vi "Measure_Synthetic_Jet.vi"(3 "Mode":T1=enum."Run VI", 5 "Traverse line In":T3={"Start X"=0.0, "Start Y"=0.0, "Start Z"=0.0, "End X"=nan, "End Y"=nan, "End Z"=nan, "No. of pts."=5, "Spacing"=enum."Linear", "Filename"=path "C:/EnFlo_Data_Local/2013/Aero_Tunnel/Nick_Martin/Results/01-2013/QA_test_I.xls", "Tunnel Speed"=nan, "Averaging time (min)"=0.08, "Extra Commands"="", "Specific Arguments"="Measure_Synthetic_Jet.vi; 200; 1000; 100", "Emission Rate (l/min)"=nan, "Trace Gas Concentration (%)"=nan, "Density Ratio"="  ---------", "Comments"="", "Row No"=0, "Row Type Selector"=enum."Run VI Named:", "Completion time"="17:12  07-01-2013", "Row Duration (mins)"=4.483248000000001, "No. of Valid pts."=5, "Meas Setup File"="LDA_SJ_A.xls"} {"Row Duration (mins)" format="%#.1f"; "Row No" min=0; "Trace Gas Concentration (%)" min=0.0 format="%#.2f"; "Emission Rate (l/min)" format="%#.2f"; "Tunnel Speed" format="%#.2f"; "Start X" format="%#.2f"; "Start Y" format="%#.2f"; "Start Z" format="%#.2f"; "End X" format="%#.2f"; "End Y" format="%#.2f"; "End Z" format="%#.2f"; "Averaging time (min)" min=0.0 format="%#.2f"}) -> (0 "Error Message":string, 1 "Status":T2, 2 "Traverse line Out":T3={"Start X"=0.0, "Start Y"=0.0, "Start Z"=0.0, "End X"=nan, "End Y"=nan, "End Z"=nan, "No. of pts."=5, "Spacing"=enum."Linear", "Filename"=path "C:/EnFlo_Data_Local/2013/Aero_Tunnel/Nick_Martin/Results/01-2013/QA_test_I.xls", "Tunnel Speed"=nan, "Averaging time (min)"=0.08, "Extra Commands"="", "Specific Arguments"="Measure_Synthetic_Jet.vi; 200; 1000; 100", "Emission Rate (l/min)"=nan, "Trace Gas Concentration (%)"=nan, "Density Ratio"="  ---------", "Comments"="", "Row No"=0, "Row Type Selector"=enum."Run VI Named:", "Completion time"="17:12  07-01-2013", "Row Duration (mins)"=4.483248000000001, "No. of Valid pts."=5, "Meas Setup File"="LDA_SJ_A.xls"} {"Row Duration (mins)" format="%#.1f"; "Row No" min=0; "Trace Gas Concentration (%)" min=0.0 format="%#.2f"; "Emission Rate (l/min)" format="%#.2f"; "Tunnel Speed" format="%#.2f"; "Start X" format="%#.2f"; "Start Y" format="%#.2f"; "Start Z" format="%#.2f"; "End X" format="%#.2f"; "End Y" format="%#.2f"; "End Z" format="%#.2f"; "Averaging time (min)" min=0.0 format="%#.2f"})   [LabVIEW 2012]
uses:
  Gen Trav/Traverse_cluster.ctl
  Gen Trav/Spacing.ctl
  Controls/Multi_run_mode.ctl
  Gen Trav/Multi_Run_Status.ctl
  Controls/User_Specific_mode.ctl
  Controls/Setup.ctl
  Controls/Save_Data.ctl
  ADAM Client/Sub VIs/ADAM Controls/Update_scan_value.ctl
  Globals/Meas_global.vi
  Globals/Synthetic_jet_global.vi
  <vilib>/Analysis/1siggen.llb/Ramp Pattern by Samples.vi
  Globals/Extra_Commands_Global.vi
  <vilib>/Analysis/NI_AALBase.lvlib
panel:
  in  "Enter SJ Data?":bool=TRUE
  in  "Stop Button":bool
  out "Last Meas Point":bool=TRUE
  out "Data":cluster{"Ramp Pattern":dbl[], dbl[]}[](graph)
  in  "Channels to Analyse":i32[](listbox)=[0]
  in  "VISA resource name":refnum<visa-resource-name>="USB0::0x0699::0x0347::C036837::INSTR"
  out "First Meas Point":bool=TRUE
  # "Check the Multirun in order to populate these Channels!"
  # "X           Y            Z"
  # "Start"
  # "End"
  # "X           Y            Z"
  # "Start"
  # "End"
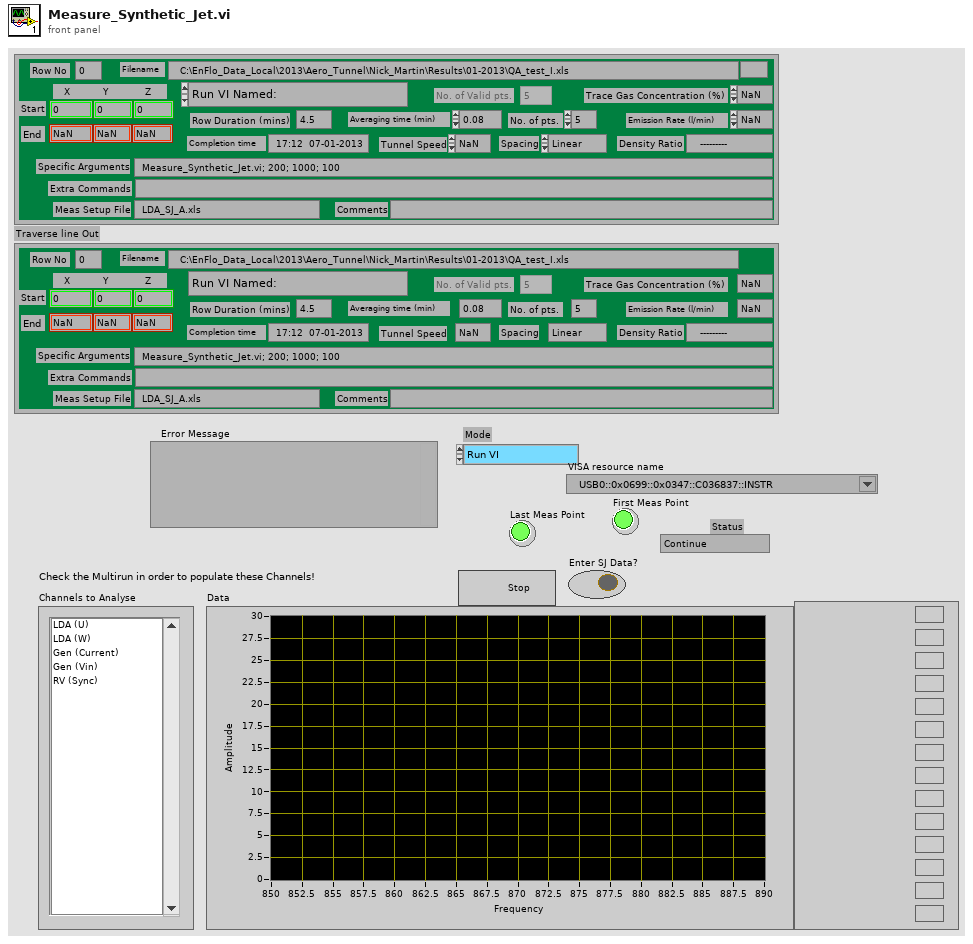
[diagram p1: front panel]
types:
  T1 = typedef "User_Specific_mode.ctl" = enum16{"Check VI only", "Run VI"}
  T2 = typedef "Multi_Run_Status.ctl" = enum16{"Continue", "Jump to Next Point", "Jump to Next Row", "Jump To Fall Back", "Terminate Run"}
  T3 = typedef "Traverse_cluster.ctl" = cluster{"Start X":dbl, "Start Y":dbl, "Start Z":dbl, "End X":dbl, "End Y":dbl, "End Z":dbl, "No. of pts.":i32, "Spacing":T4, "Filename":path, "Tunnel Speed":dbl, "Averaging time (min)":dbl, "Extra Commands":string, "Specific Arguments":string, "Emission Rate (l/min)":dbl, "Trace Gas Concentration (%)":dbl, "Density Ratio":string, "Comments":string, "Row No":i32, "Row Type Selector":T5, "Completion time":string, "Row Duration (mins)":dbl, "No. of Valid pts.":i32, "Meas Setup File":string}
  T4 = typedef "Spacing.ctl" = enum16{"Linear", "Log", "Gauss", "Specified", "N/A"}
  T5 = typedef "Multi_run_mode.ctl" = enum16{"Move Traverse Only", "Set Tunnel Speed Only", "Set Source Only", "Set Measurement Conditions", "Single Measurement", "Vertical Profile", "Lateral Profile", "Longitudinal Profile", "Explore Volume", "Multi-Axis Profile", "Auto Calibrate", "Meas Fast FID Bkgnd", "Check Beam Power", "Scanning Valve Measurement", "Run VI Named:", "Set ADAM Ch", "Wait (minutes)", "Send Message", "Synchronize With:", "Fall Back to this Row", "Turn Off Row Repeating", "Blank Row", "Traverse 3D Volume"}
  T6 = typedef "Analysis_info_cluster.ctl" = cluster{"Colour":u32, "Inst type":T7, "Inst name":string, "Symbol":string, "Code name":string, "Extra Info":string, "Inst Array":T8, "Extra Titles":string[], "Extra Values":string[], "U":dbl, "u^2":dbl, "u^3":dbl, "u^4":dbl, "Skew_u":dbl, "Kurt_u":dbl, "Sd Error in Mean":dbl, "% u'/U":dbl, "X":dbl, "Y":dbl, "Z":dbl, "Timescale integral to 25%":dbl, "Sd Error in Variance":dbl, "Calib File":path, "Calib Constants":dbl[], "Output Position":bool, "Full Stats":bool, "Av Sampling Rate":dbl, "Av No of Samples":dbl, "Total Meas Time (s)":dbl, "ADAM Ch Name":string}
  T7 = typedef "Inst_type.ctl" = enum16{"Propeller anemometer", "Raw voltage", "Pressure Transducer", "Pitot-static tube", "Preston tube", "Hot wire", "Cross wire 1", "Cross wire 2", "Generic Linear", "Generic Polynomial", "Generic BackPoly", "Fast FID", "Thermocouple", "Cold wire", "Pulsed Wire", "LDA Vel", "LDA Tran time", "LDA Arr time"}
  T8 = typedef "Instrument_Array.ctl" = enum16{"PWA", "LDA", "Analogue"}
  T9 = typedef "Save_Data.ctl" = enum16{"Save No Data", "Save Data"}
  T10 = typedef "Setup.ctl" = enum16{"Run Program", "Show Setup", "Save Current Setup", "Setup Front Panel"}
  T11 = typedef "SJ_Data_Cluster.ctl" = cluster{"Do (mm)":dbl, "Dc (mm)":dbl, "Ho (mm)":dbl, "Hc (mm)":dbl, "K":dbl, "beta":dbl, "Vc (m^3)":dbl, "Vo (m^3)":dbl}
  T12 = typedef "Update_scan_value.ctl" = cluster{"Channel Name":string, "New Value":dbl}
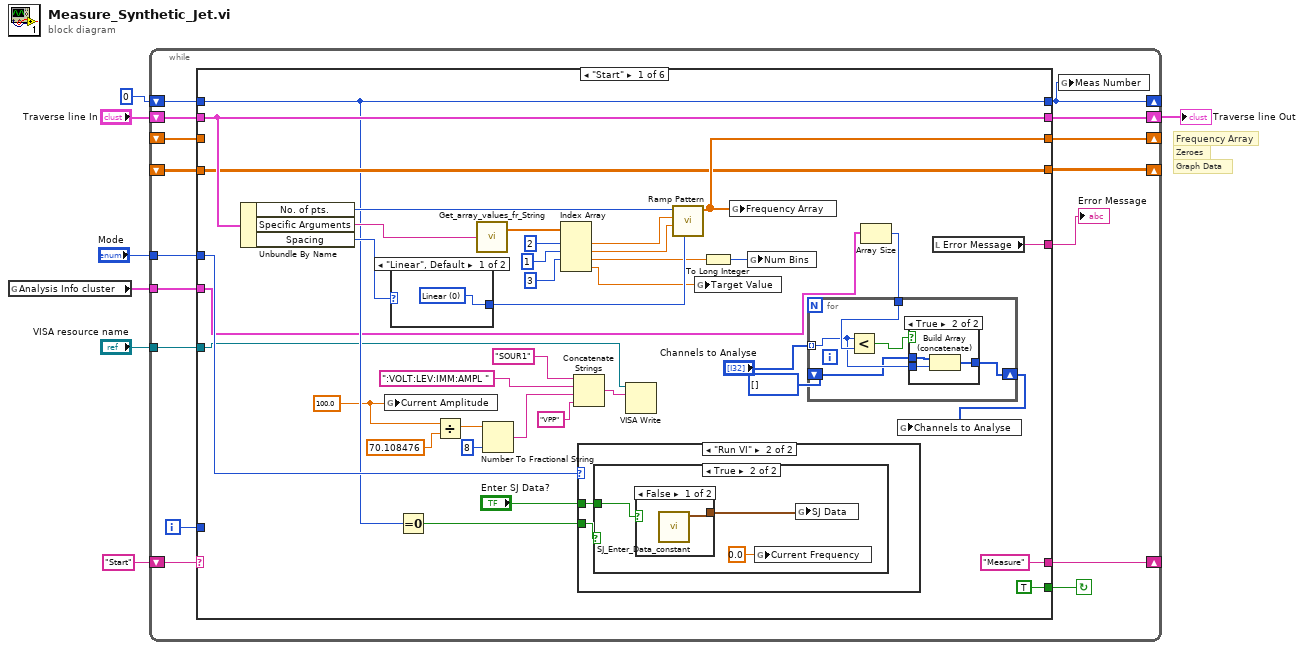
[diagram p0: block diagram]
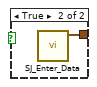
[diagram p5: hidden frame]
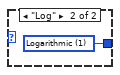
[diagram p6: hidden frame]
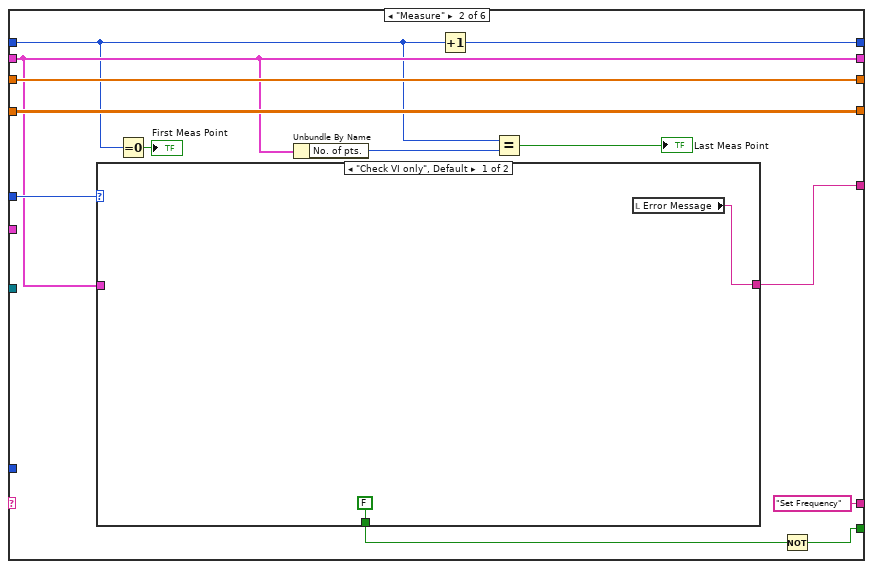
[diagram p7: hidden frame]
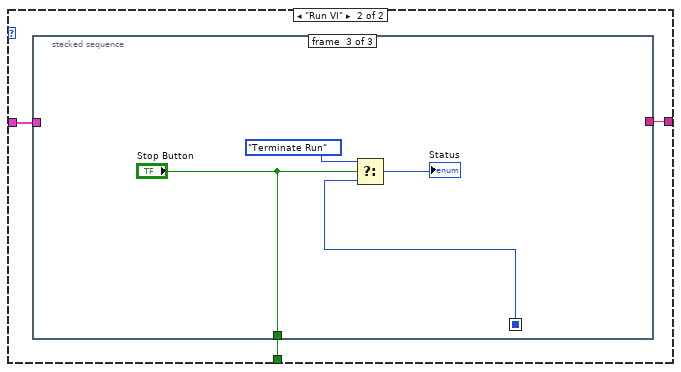
[diagram p8: hidden frame]
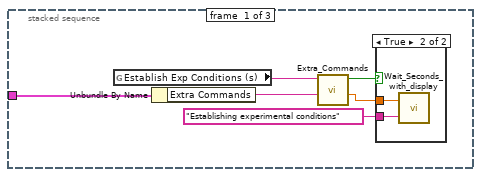
[diagram p9: hidden frame]
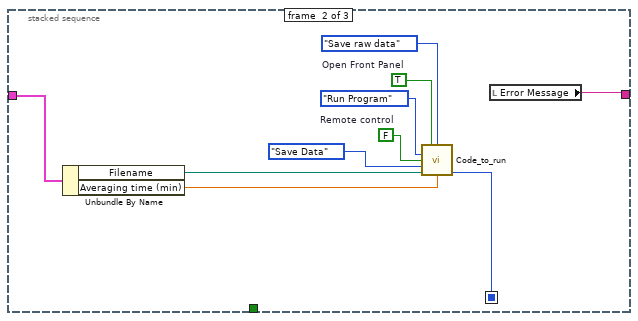
[diagram p11: hidden frame]
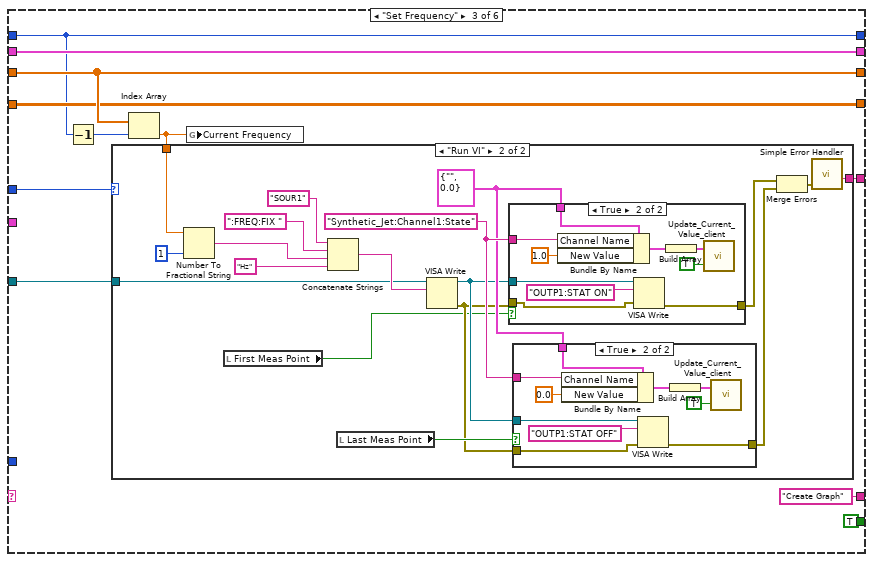
[diagram p12: hidden frame]
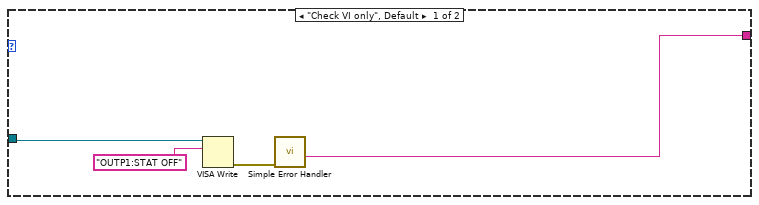
[diagram p13: hidden frame]
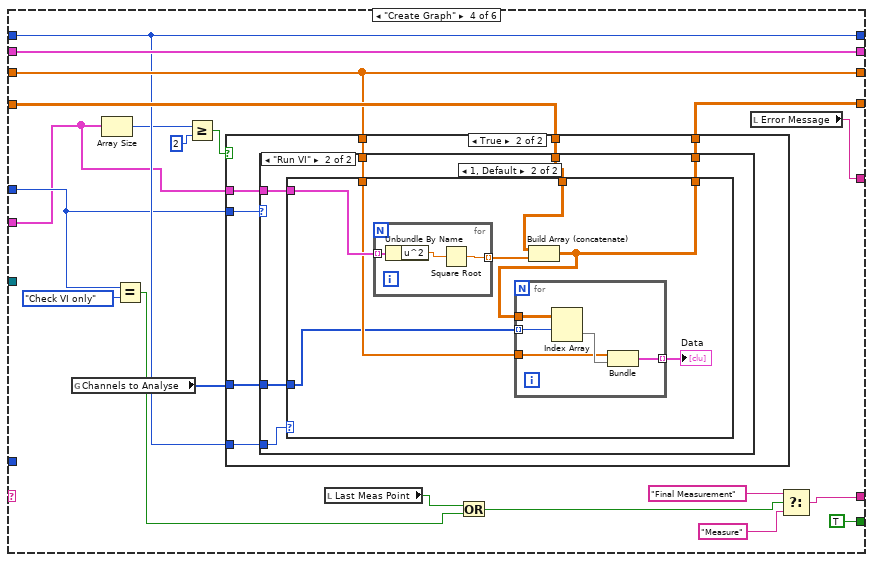
[diagram p16: hidden frame]
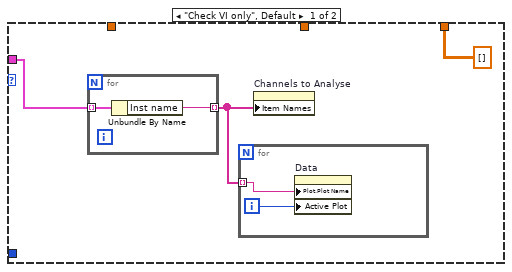
[diagram p18: hidden frame]
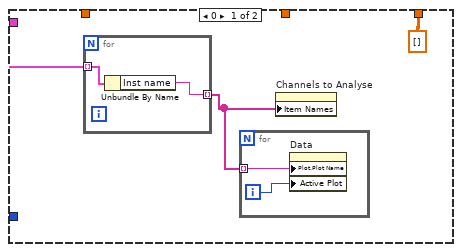
[diagram p19: hidden frame]
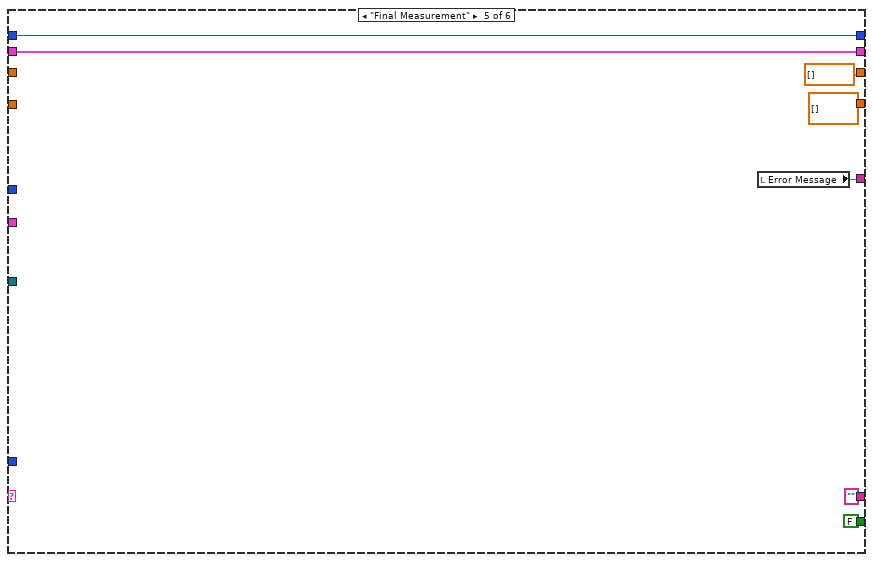
[diagram p20: hidden frame]
diagram:
  # "Graph Data"
  # "Zeroes"
  # "Frequency Array"
  n1 = global read "Meas_global.vi" "Analysis Info cluster"() -> (w1:T6[])
  n2 = while {
    shift-right: [w21] -> _
    shift-left: "Start" -> [w20]
    shift-right: [w19] -> w5
    shift-left: "Traverse line In" -> [w23]
    shift-right: [w18] -> _
    shift-left: _ -> [w17]
    tunnel: "Mode" -> [w16]
    tunnel: "VISA resource name" -> [w14]
    shift-right: [w13] -> _
    shift-left: _ -> [w12]
    shift-right: [w9] -> _
    shift-left: 0 -> [w10]
    tunnel: w1 -> [w8]
    i -> [w15]
    stop <- w22 continue-if-true
    n3 = case shown="\"Start\"" w20 {
      selector: w20 -> [_ _ _ _ _ w249]
      tunnel: w23 -> [w59 w86 w128 w194 w242 w257]
      tunnel: [TRUE w80 TRUE TRUE ("Last Meas Point") FALSE ("Last Meas Point") FALSE] -> w22
      tunnel: ["Measure" "Set Frequency" "Create Graph" w188 "" ""] -> w21
      tunnel: [w59 w86 w128 w194 w242 w257] -> w19
      tunnel: [w47 w91 w127 w191 dbl[] [] ("Ramp Pattern") w248] -> w18
      tunnel: w17 -> [_ w91 w127 w191 _ w248]
      tunnel: w16 -> [w48 w90 w123 w184 _ _]
      tunnel: w15 -> [_ _ _ _ _ _]
      tunnel: w14 -> [w33 _ w124 _ _ _]
      tunnel: [w46 w89 w122 w193 dbl[][] [] w247] -> w13
      tunnel: w12 -> [w46 w89 w122 w192 _ w247]
      tunnel: [w45 w88 w121 w190 w241 w246] -> w11
      tunnel: [w41 w84 w120 w185 w238 w245] -> w9
      tunnel: w10 -> [w41 w82 w120 w185 w238 w245]
      tunnel: w8 -> [w28 _ _ w175 _ _]
      frame "Start" {
        w30 = 100.0 ("number")
        n4 = Unbundle By Name(w59) -> ("No. of pts."=w58:i32, "Specific Arguments"=w55:string, "Spacing"=w57:T4)
        n5 = global write "Synthetic_jet_global.vi" "Current Amplitude"(w30) -> ()
        n6 = case shown="\"Linear\", Default" w57 {
          tunnel: [w78 w79] -> w56
          frame "Linear", Default {
            w78 = u16 0 items=["Linear", "Logarithmic"] ("type")
          }
          frame "Log" {
            w79 = u16 1 items=["Linear", "Logarithmic"] ("type")
          }
        }
        n7 = Equal To 0?(x=w41) -> (x = 0?=w49:bool)
        n8 = Divide(x=w30, y=70.108476) -> (x/y=w32:dbl)
        n9 = call "Get_array_values_fr_String.vi"("String Value"=w55) -> ("Numeric Array"=w54:dbl[])  [unwired: 1 out]
        n10 = Number To Fractional String(number=w32, precision (6)=i16 8) -> (F-format string=w35:string)  [unwired: 2 in]
        n11 = Index Array(array=w54, index #1=2 ("index"), index #2=1 ("index"), index #3=3 ("index")) -> (element #1=w51:dbl, element #2=w50:dbl, element #3=w43:dbl, element #4=w40:dbl)  [unwired: 1 in]
        n12 = Concatenate Strings("SOUR1" ("string"), ":VOLT:LEV:IMM:AMPL " ("string"), w35, "VPP" ("string")) -> (w36:string)
        n13 = case shown="\"Run VI\"" w48 {
          tunnel: w49 -> [_ w72]
          tunnel: "Enter SJ Data?" -> [_ w71]
          frame "Check VI only", Default {
          }
          frame "Run VI" {
            n14 = case shown="True" w72 {
              tunnel: w71 -> [_ w74]
              frame False {
              }
              frame True {
                n15 = case shown="False" w74 {
                  tunnel: [w76 w77] -> w73
                  frame False {
                    n16 = call "SJ_Enter_Data_constant.vi"() -> ("SJ Data"=w76:T11)  [unwired: 11 in]
                  }
                  frame True {
                    n17 = call "SJ_Enter_Data.vi"() -> ("SJ Data"=w77:T11)  [unwired: 11 in]
                  }
                }
                n18 = global write "Synthetic_jet_global.vi" "Current Frequency"(0.0 ("Current Frequency")) -> ()
                n19 = global write "Synthetic_jet_global.vi" "SJ Data"(w73) -> ()
              }
            }
          }
        }
        n20 = VISA Write(VISA resource name=w33, write buffer=w36) -> ()  [unwired: 1 in, 3 out]
        n21 = call-poly <vilib>:"Ramp Pattern.vi"("type"=w56, "start"=w50, "end"=w51, "samples"=w58) -> ("Ramp Pattern"=w47:dbl[])  [unwired: 6 in, 1 out]
        n22 = global write "Synthetic_jet_global.vi" "Target Value"(w40) -> ()
        n23 = To Long Integer(number=w43) -> (32bit integer=w42:i32)
        n24 = global write "Synthetic_jet_global.vi" "Frequency Array"(w47) -> ()
        n25 = global write "Synthetic_jet_global.vi" "Num Bins"(w42) -> ()
        n26 = Array Size(array=w28) -> (size(s)=w29:i32)
        n27 = for {
          tunnel: w29 -> [w66]
          tunnel: "Channels to Analyse" -> [w64] mode=indexing
          shift-right: [w63] -> w26
          shift-left: i32[] [] -> [w62]
          n28 = Less?(x=w64, y=w66) -> (x < y?=w65:bool)
          n29 = case shown="True" w65 {
            tunnel: w64 -> [_ w70]
            tunnel: [w67 w69] -> w63
            tunnel: w62 -> [w67 w68]
            frame False {
            }
            frame True {
              n30 = Build Array (concatenate)(w68, w70) -> (w69:i32[])
            }
          }
        }
        n31 = global write "Synthetic_jet_global.vi" "Channels to Analyse"(w26) -> ()
        n32 = local read "Error Message"() -> (w45:string)
      }
      frame "Measure" {
        n33 = case shown="\"Check VI only\", Default" w90 {
          tunnel: w86 -> [_ w97]
          tunnel: [w94 w96] -> w88
          tunnel: [FALSE ("Stop Button") w95] -> w81
          frame "Check VI only", Default {
            n34 = local read "Error Message"() -> (w94:string)
          }
          frame "Run VI" {
            n35 = stacked-sequence {
              seq-local: [_ w106 _] -> [_ _ w117]
              tunnel: w97 -> [w98 w111 _]
              tunnel: [_ w108 _] -> w96
              tunnel: [_ _ "Stop Button"] -> w95
              frame #0 {
                n36 = global read "Extra_Commands_Global.vi" "Establish Exp Conditions (s)"() -> (w101:string)
                n37 = Unbundle By Name(w98) -> ("Extra Commands"=w99:string)
                n38 = call "Extra_Commands.vi"("String to Search"=w99, "Command"=w101) -> ("Numeric Value"=w100:dbl, "Command Found"=w102:bool)  [unwired: 2 in, 2 out]
                n39 = case shown="True" w102 {
                  tunnel: w100 -> [_ w105]
                  tunnel: "Establishing experimental conditions" ("Message") -> [_ w104]
                  frame False {
                  }
                  frame True {
                    n40 = call "Wait_Seconds_with_display.vi"("Message"=w104, "Seconds to wait"=w105) -> ()  [unwired: 1 in, 1 out]
                  }
                }
              }
              frame #1 {
                w113 = TRUE  # Open Front Panel
                w112 = FALSE  # Remote control
                n41 = Unbundle By Name(w111) -> ("Filename"=w110:path, "Averaging time (min)"=w107:dbl)
                n42 = call "Code_to_run.vi"("Open Front Panel"=w113, "Raw data option"=enum16{"Save raw data", "Raw data not saved"}."Save raw data", "setup"=Setup."Run Program", "Remote control"=w112, "File"=Save_Data."Save Data", "Results Filename"=w110, "Averaging time (min)"=w107) -> ("Status"=w106:T2)  [unwired: 4 in, 4 out]
                n43 = local read "Error Message"() -> (w108:string)
              }
              frame #2 {
                n44 = Select(t=Multi_Run_Status."Terminate Run", s="Stop Button", f=w117) -> (s? t:f=→"Status":T2)
              }
            }
          }
        }
        n45 = Equal To 0?(x=w82) -> (x = 0?=→"First Meas Point":bool)
        n46 = Unbundle By Name(w86) -> ("No. of pts."=w85:i32)
        n47 = Increment(x=w82) -> (x+1=w84:i32)
        n48 = Equal?(x=w82, y=w85) -> (x = y?=→"Last Meas Point":bool)
        n49 = Not(x=w81) -> (.not. x?=w80:bool)
      }
      frame "Set Frequency" {
        n50 = Decrement(x=w120) -> (x-1=w126:i32)
        n51 = Index Array(array=w127, index=w126) -> (element=w125:dbl)
        n52 = case shown="\"Run VI\"" w123 {
          tunnel: w125 -> [_ w144]
          tunnel: w124 -> [w133 w143]
          tunnel: [w131 w140] -> w121
          frame "Check VI only", Default {
            n53 = VISA Write(VISA resource name=w133, write buffer="OUTP1:STAT OFF") -> (error out=w132:errorcluster)  [unwired: 1 in, 2 out]
            n54 = call <vilib>:"Simple Error Handler.vi"("error in (no error)"=w132) -> ("source out"=w131:string)  [unwired: 4 in, 4 out]
          }
          frame "Run VI" {
            w145 = T12 {"Channel Name"="", "New Value"=0.0} ("Update Scan Value Cluster")
            w146 = "Synthetic_Jet:Channel1:State" ("write buffer")
            n55 = Number To Fractional String(number=w144, precision (6)=i16 1) -> (F-format string=w150:string)  [unwired: 2 in]
            n56 = local read "First Meas Point"() -> (w135:bool)
            n57 = Concatenate Strings("SOUR1", ":FREQ:FIX " ("string"), w150, "Hz" ("string")) -> (w152:string)
            n58 = local read "Last Meas Point"() -> (w142:bool)
            n59 = VISA Write(VISA resource name=w143, write buffer=w152) -> (VISA resource name out=w141:refnum<visa-resource-name>, error out=w136:errorcluster)  [unwired: 1 in, 1 out]
            n60 = case shown="True" w135 {
              tunnel: w146 -> [_ w169]
              tunnel: w145 -> [_ w168]
              tunnel: w141 -> [_ w167]
              tunnel: [w164 w166] -> w137
              tunnel: w136 -> [w164 w165]
              frame False {
              }
              frame True {
                n61 = Bundle By Name(cluster=w168, "Channel Name"=w169, "New Value"=1.0) -> (w172:T12)
                n62 = VISA Write(VISA resource name=w167, write buffer="OUTP1:STAT ON", error in (no error)=w165) -> (error out=w166:errorcluster)  [unwired: 2 out]
                n63 = Build Array(w172) -> (w171:T12[])
                n64 = call "Update_Current_Value_client.vi"("Don't Bother with check?"=TRUE, "Update array in"=w171) -> ()
              }
            }
            n65 = case shown="True" w142 {
              tunnel: w146 -> [_ w158]
              tunnel: w145 -> [_ w157]
              tunnel: w141 -> [_ w156]
              tunnel: [w153 w155] -> w138
              tunnel: w136 -> [w153 w154]
              frame False {
              }
              frame True {
                n66 = Bundle By Name(cluster=w157, "Channel Name"=w158, "New Value"=0.0) -> (w161:T12)
                n67 = VISA Write(VISA resource name=w156, write buffer="OUTP1:STAT OFF", error in (no error)=w154) -> (error out=w155:errorcluster)  [unwired: 2 out]
                n68 = Build Array(w161) -> (w160:T12[])
                n69 = call "Update_Current_Value_client.vi"("Don't Bother with check?"=TRUE, "Update array in"=w160) -> ()
              }
            }
            n70 = Merge Errors(w137, w138) -> (w139:errorcluster)
            n71 = call <vilib>:"Simple Error Handler.vi"("error in (no error)"=w139) -> ("source out"=w140:string)  [unwired: 4 in, 4 out]
          }
        }
        n72 = global write "Synthetic_jet_global.vi" "Current Frequency"(w125) -> ()
      }
      frame "Create Graph" {
        n73 = global read "Synthetic_jet_global.vi" "Channels to Analyse"() -> (w176:i32[])
        n74 = Array Size(array=w175) -> (size(s)=w177:i32)
        n75 = Equal?(x=w184, y=User_Specific_mode."Check VI only") -> (x = y?=w181:bool)
        n76 = Greater Or Equal?(x=w177, y=2 ("x")) -> (x >= y?=w179:bool)
        n77 = case shown="True" w179 {
          tunnel: w175 -> [_ w202]
          tunnel: [w195 w201] -> w193
          tunnel: w192 -> [w195 w200]
          tunnel: w191 -> [_ w199]
          tunnel: w185 -> [_ w198]
          tunnel: w184 -> [_ w197]
          tunnel: w176 -> [_ w196]
          frame False {
          }
          frame True {
            n78 = case shown="\"Run VI\"" w197 {
              tunnel: w202 -> [w205 w215]
              tunnel: w198 -> [_ w214]
              tunnel: [dbl[][] [] w213] -> w201
              tunnel: w200 -> [_ w212]
              tunnel: w199 -> [_ w211]
              tunnel: w196 -> [_ w210]
              frame "Check VI only", Default {
                n79 = for {
                  tunnel: w205 -> [w209] mode=indexing
                  tunnel: [w208] -> w203 mode=indexing
                  n80 = Unbundle By Name(w209) -> ("Inst name"=w208:string)
                }
                n81 = for {
                  tunnel: w203 -> [w207] mode=indexing
                  i -> [w206]
                  n82 = property on="Data" class="XYGraph (strict)"("Plot.Plot Name"=w207, "Active Plot"=w206) -> ()  [unwired: 2 in, 2 out]
                }
                n83 = property on="Channels to Analyse" class="LstBox (strict)"("Item Names"=w203) -> ()  [unwired: 2 in, 2 out]
              }
              frame "Run VI" {
                n84 = case shown="1, Default" w214 {
                  tunnel: w215 -> [w218 w229]
                  tunnel: [dbl[][] [] w226] -> w213
                  tunnel: w212 -> [_ w227]
                  tunnel: w211 -> [_ w225]
                  tunnel: w210 -> [_ w223]
                  frame 0 {
                    n85 = for {
                      tunnel: w218 -> [w222] mode=indexing
                      tunnel: [w221] -> w216 mode=indexing
                      n86 = Unbundle By Name(w222) -> ("Inst name"=w221:string)
                    }
                    n87 = for {
                      tunnel: w216 -> [w220] mode=indexing
                      i -> [w219]
                      n88 = property on="Data" class="XYGraph (strict)"("Plot.Plot Name"=w220, "Active Plot"=w219) -> ()  [unwired: 2 in, 2 out]
                    }
                    n89 = property on="Channels to Analyse" class="LstBox (strict)"("Item Names"=w216) -> ()  [unwired: 2 in, 2 out]
                  }
                  frame 1, Default {
                    n90 = for {
                      tunnel: w229 -> [w237] mode=indexing
                      tunnel: [w235] -> w228 mode=indexing
                      n91 = Unbundle By Name(w237) -> ("u^2"=w236:dbl)
                      n92 = Square Root(x=w236) -> (sqrt(x)=w235:dbl)
                    }
                    n93 = Build Array (concatenate)(w227, w228) -> (w226:dbl[][])
                    n94 = for {
                      tunnel: w226 -> [w234]
                      tunnel: w223 -> [w230] mode=indexing
                      tunnel: w225 -> [w232]
                      tunnel: [w231] -> w224 mode=indexing
                      n95 = Index Array(array=w234, index (row)=w230) -> (element=w233:dbl[])  [unwired: 1 in]
                      n96 = Bundle("Ramp Pattern"=w232, w233) -> (w231:cluster{"Ramp Pattern":dbl[], dbl[]})  [unwired: 1 in]
                    }
                    "Data" <- w224
                  }
                }
              }
            }
          }
        }
        n97 = local read "Last Meas Point"() -> (w182:bool)
        n98 = Or(x=w182, y=w181) -> (x .or. y?=w180:bool)
        n99 = local read "Error Message"() -> (w190:string)
        n100 = Select(t="Final Measurement", s=w180, f="Measure") -> (s? t:f=w188:string)
      }
      frame "Final Measurement" {
        n101 = local read "Error Message"() -> (w241:string)
      }
      frame "No Match", Default {
        n102 = Current VI's Path() -> (path=w254:path)
        n103 = Format Into String(format string="The Case\"%s\" was not Matched\nin VI named\n'%s\"" ("Format String"), w249, w254) -> (resulting string=w251:string)  [unwired: 2 in, 1 out]
        n104 = One Button Dialog(message=w251, button name ("OK")="STOP") -> (true=w253:bool)
        n105 = Stop(stop? (T)=w253) -> ()
        n106 = local read "Error Message"() -> (w246:string)
      }
    }
    "Error Message" <- w11
    n107 = global write "Synthetic_jet_global.vi" "Meas Number"(w9) -> ()
  }
  "Traverse line Out" <- w5
